vi "Control_ControPIDEvent.vi"(8 "error in":errorcluster, 9 "array_enc_in":T1, 10 "Estado":T6, 11 "New_data?":bool) -> (0 "error out":errorcluster, 2 "Cluster_Dashboard":refnum<user-event>)   [LabVIEW 2026]
uses:
  Control/Ctrl_ControlPIDEvent.ctl
  Control/Ctrl_Dashboard_StateMach.ctl
  Control/Ctrl_Errores.ctl
  Control/Ctrl_Motores_Valores.ctl
  Control/Ctrl_datos6motores_final.ctl
  Control/Ctr_Enc_Values.ctl
  Control/Ctrl_Array_Enc_Out.ctl
  Control/Cluster_Dashboard.ctl
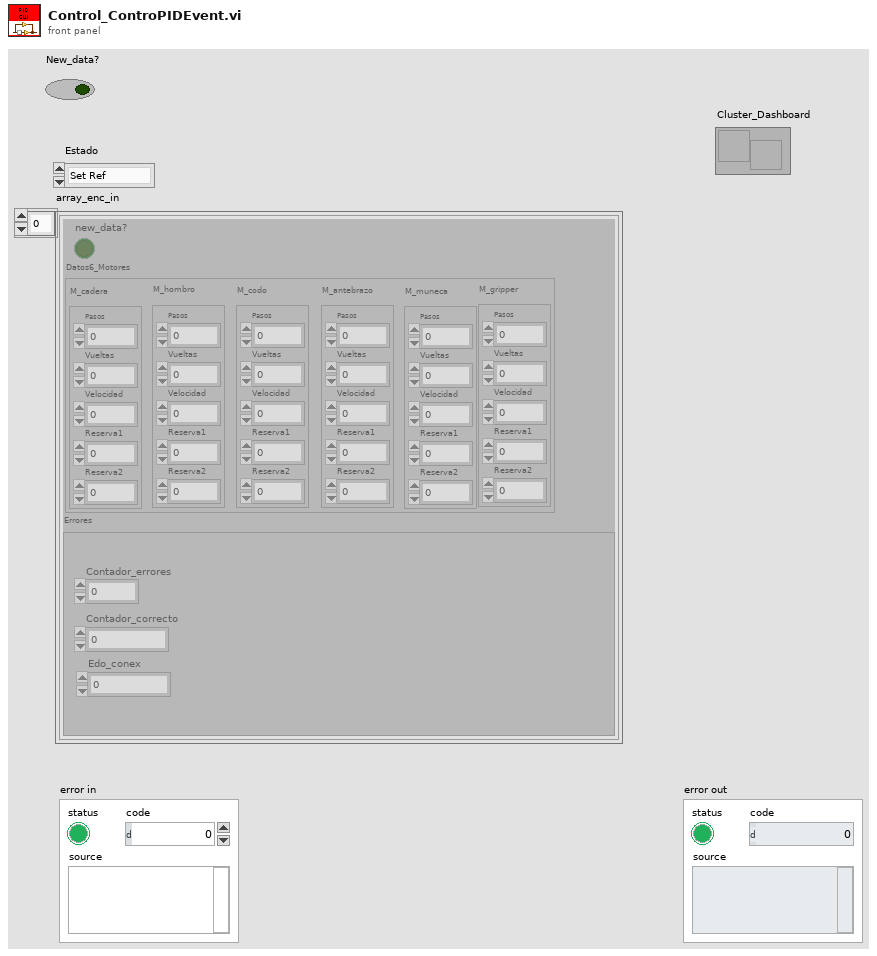
[diagram p1: front panel]
types:
  T1 = typedef "Ctrl_Array_Enc_Out.ctl" = T2[]
  T2 = typedef "Ctr_Enc_Values.ctl" = cluster{"Datos6_Motores":T3, "Errores":T5, "new_data?":bool}
  T3 = typedef "Ctrl_datos6motores_final.ctl" = cluster{"M_cadera":T4, "M_hombro":T4, "M_codo":T4, "M_antebrazo":T4, "M_muneca":T4, "M_gripper":T4}
  T4 = typedef "Ctrl_Motores_Valores.ctl" = cluster{"Pasos":i32, "Vueltas":i16, "Velocidad":dbl, "Reserva1":u8, "Reserva2":u8}
  T5 = typedef "Ctrl_Errores.ctl" = cluster{"Contador_correcto":u32, "Contador_errores":u32, "Edo_conex":u32}
  T6 = typedef "Ctrl_ControlPIDEvent.ctl" = enum16{"Set Ref", "Update Enc", "Stop", "Get Ref"}
  T7 = typedef "Cluster_Dashboard.ctl" = cluster{"Array_encoders":T1, "Estado":T8}
  T8 = typedef "Ctrl_Dashboard_StateMach.ctl" = enum16{"Stop", "Update", "Start"}
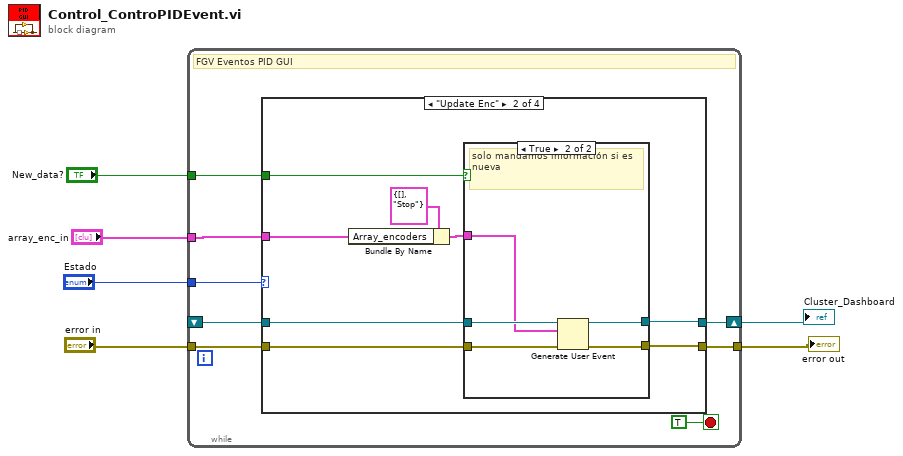
[diagram p0: block diagram]
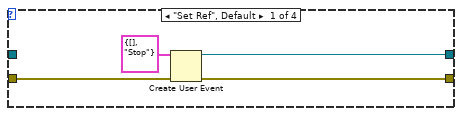
[diagram p2: hidden frame]
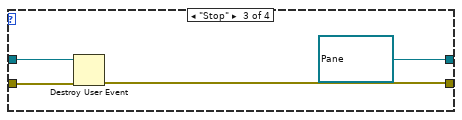
[diagram p4: hidden frame]
diagram:
  n1 = while {
    tunnel: "error in" -> [w13]
    tunnel: "Estado" -> [w14]
    tunnel: [w12] -> w4
    shift-right: [w10] -> w1
    shift-left: _ -> [w9]
    tunnel: "array_enc_in" -> [w7]
    tunnel: "New_data?" -> [w8]
    stop <- TRUE stop-if-true
    # "FGV Eventos PID GUI"
    n2 = case shown="\"Update Enc\"" w14 {
      tunnel: w13 -> [w18 w22 w37 w39]
      tunnel: [w17 w23 w36 w39] -> w12
      tunnel: [w16 w24 refnum<user-event> refnum ("Cluster_Dashboard") w38] -> w10
      tunnel: w9 -> [_ w21 w35 w38]
      tunnel: w8 -> [_ w19 _ _]
      tunnel: w7 -> [_ w20 _ _]
      frame "Set Ref", Default {
        n3 = Create User Event(user event datatype=T7 {"Array_encoders"=[], "Estado"=enum."Stop"} ("Cluster_Dashboard"), error in=w18) -> (user event=w16:refnum<user-event>, error out=w17:errorcluster)
      }
      frame "Update Enc" {
        n4 = Bundle By Name(cluster=T7 {"Array_encoders"=[], "Estado"=enum."Stop"}, "Array_encoders"=w20) -> (w25:T7)
        n5 = case shown="True" w19 {
          tunnel: w22 -> [w28 w33]
          tunnel: [w28 w32] -> w23
          tunnel: w25 -> [_ w29]
          tunnel: w21 -> [w27 w31]
          tunnel: [w27 w30] -> w24
          frame False {
            # "no hay información nueva"
          }
          frame True {
            # "solo mandamos información si es nueva"
            n6 = Generate User Event(user event=w31, event data cluster=w29, error in=w33) -> (user event out=w30:refnum<user-event>, error out=w32:errorcluster)  [unwired: 1 in]
          }
        }
      }
      frame "Stop" {
        n7 = Destroy User Event(user event=w35, error in=w37) -> (error out=w36:errorcluster)
      }
      frame "Get Ref" {
      }
    }
  }
  "error out" <- w4
  "Cluster_Dashboard" <- w1
